vi "REPORT_OPRTN_reformat_reals.vi"(11 "reals_in":string[](array[string])) -> (3 "reals_out":string[](array[string]))   [LabVIEW 2019]
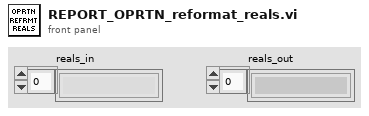
[diagram p1: front panel]
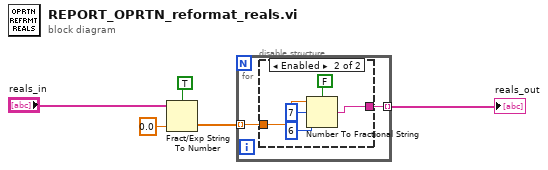
[diagram p0: block diagram]
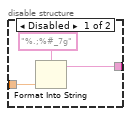
[diagram p2: hidden frame]
diagram:
  n1 = Fract/Exp String To Number(use system decimal point (T)=TRUE, string="reals_in", default (0 dbl)=sgl 0.0 ("default (0 DBL)")) -> (number=w1:sgl[])  [unwired: 1 in, 1 out]
  n2 = for {
    tunnel: w1 -> [w7] mode=indexing
    tunnel: [w6] -> w4 mode=indexing
    n3 = disable-structure shown="Enabled" {
      disable-tunnel: w7 -> [w9 w15]
      disable-tunnel: [w8 w14] -> w6
      frame Disabled {
        n4 = Format Into String(format string="%.;%#_7g", w9) -> (resulting string=w8:string)  [unwired: 2 in, 1 out]
      }
      frame Enabled {
        n5 = Number To Fractional String(use system decimal point (T)=FALSE, number=w15, width (-)=i16 7, precision (6)=i16 6) -> (F-format string=w14:string)
      }
    }
  }
  "reals_out" <- w4
